vi "Basic.vi"() -> ()   [LabVIEW 2021, in "GettingStarted_5745_Host.lvlib"]
uses:
  GettingStarted_5745_Host.lvlib
  <vilib>/userdefined/High Color/nirio_resource_hc.ctl
  <instrlib>/FlexRIO/API/Host/v1/NI FlexRIO/API/Reference Clock Source.ctl
  <vilib>/rvi/interface/common/niFpgaWaitOnOcc.vi
  <vilib>/Utility/error.llb/Error Cluster From Error Code.vi
  <instrlib>/FlexRIO/API/Host/v1/NI FlexRIO/API/Configure Reference Clock.vi
  <instrlib>/FlexRIO/API/Host/v1/NI FlexRIO/API/Configure Digital Edge Start Trigger.vi
  <instrlib>/FlexRIO/API/Host/v1/NI FlexRIO/API/Configure Immediate Start Trigger.vi
  <instrlib>/_niInstr/Streaming/v1/Host/Public/Start Continuous Stream.vi
  <vilib>/FPGAPlugInAG/Dynamic/niLvFpga_Close_Dynamic.vi
  <vilib>/rvi/interface/nirviMethod/nirviMethod.xnode
  <vilib>/rvi/interface/nirviCloseFPGA/nirviCloseFPGA.xnode
  <instrlib>/FlexRIO/API/Host/v1/NI FlexRIO API v1.lvlib
  <instrlib>/_niInstr/Streaming/v1/Host/niInstr Streaming v1 Host.lvlib
  <vilib>/FPGAPlugInAG/Dynamic/niLvFpga_ConfigureFifo_Dynamic.vi
  <vilib>/rvi/errors/niLvFpgaMergeErrorWithErrorCode.vi
panel:
  in  "reference clock source":T1 items=["Default", "Onboard", "PXI_Clk10", "External", "None", "Baseboard Reference"]
  in  "Download AO Waveforms":bool
  out "AO Out":waveform(dbl)[](graph) caption="Waveform Graph"
  in  "Phase (Deg)":dbl format="%.2p"
  in  "Phase (Deg) 2":dbl=-90.0 format="%.2p"
  in  "Enable DAC Digital Upconverter":bool
  in  "DAC Digital Upconverter Channel":string="AO0"
  in  "Amplitude (V)":dbl=0.4 format="%0.2p"
  in  "Frequency (Hz)":dbl=5000000.0 format="%0.2p"
  in  "Amplitude (V) 2":dbl=0.4 format="%0.2p"
  in  "Frequency (Hz) 2":dbl=10000000.0 format="%0.2p"
  in  "Sampling Info":cluster{"Fs":dbl, "#s":dbl}={"Fs"=3200000000.0, "#s"=3200.0} {"#s" format="%_9g"; "Fs" format="%#_6p"}
  out "Device Power":dbl(slide)=17.86 scale=-1.0..38.0 scale format="%#_3p"
  out "FPGA Temperature":dbl(slide)=45.0 scale=0.0..100.0 scale format="%#_3p"
  in  "Trigger Type":enum32{"Immediate", "Digital"}(tab)
  in  "digital trigger source":string(combo)
  in  "stop":bool
  in  "Bitfile path":path=path "C:/Program Files (x86)/National Instruments/LabVIEW 2022/ProjectTemplates/Source/FlexRIO/NI5745/Getting Started/FPGA Bitfiles/PXIe_5745_KU040.lvbitx"
  out "error out":errorcluster
  out "Limit (W)":dbl=38.0
  out "Power (W)":dbl=17.86
  out "Limit (C)":dbl=96.0
  out "Temp (C)":dbl=45.0 format="%#_4p"
  in  "RIO Device":T2="5745_1"
  # "Overview: Configure an acquisition for a FlexRIO target and transfer the data to the host using the FlexRIO Host API.  Loop an output waveform\nRequirements: FlexRIO\nInstructions: \n 1. Select the RIO Device that corresponds to the FlexRIO target. \n 2. Select the bitfile path that corresponds to your device\n 3. Optionally configure the clocking, stream, and trigger. \n 4. Run the VI"
  # "Resource Configuration"
  # "Clocking configuration"
  # "25600.0000\n22400"
  # "Output Waveform Configuration"
  # "Device Monitoring"
  # "AO 0"
  # "AO 1"
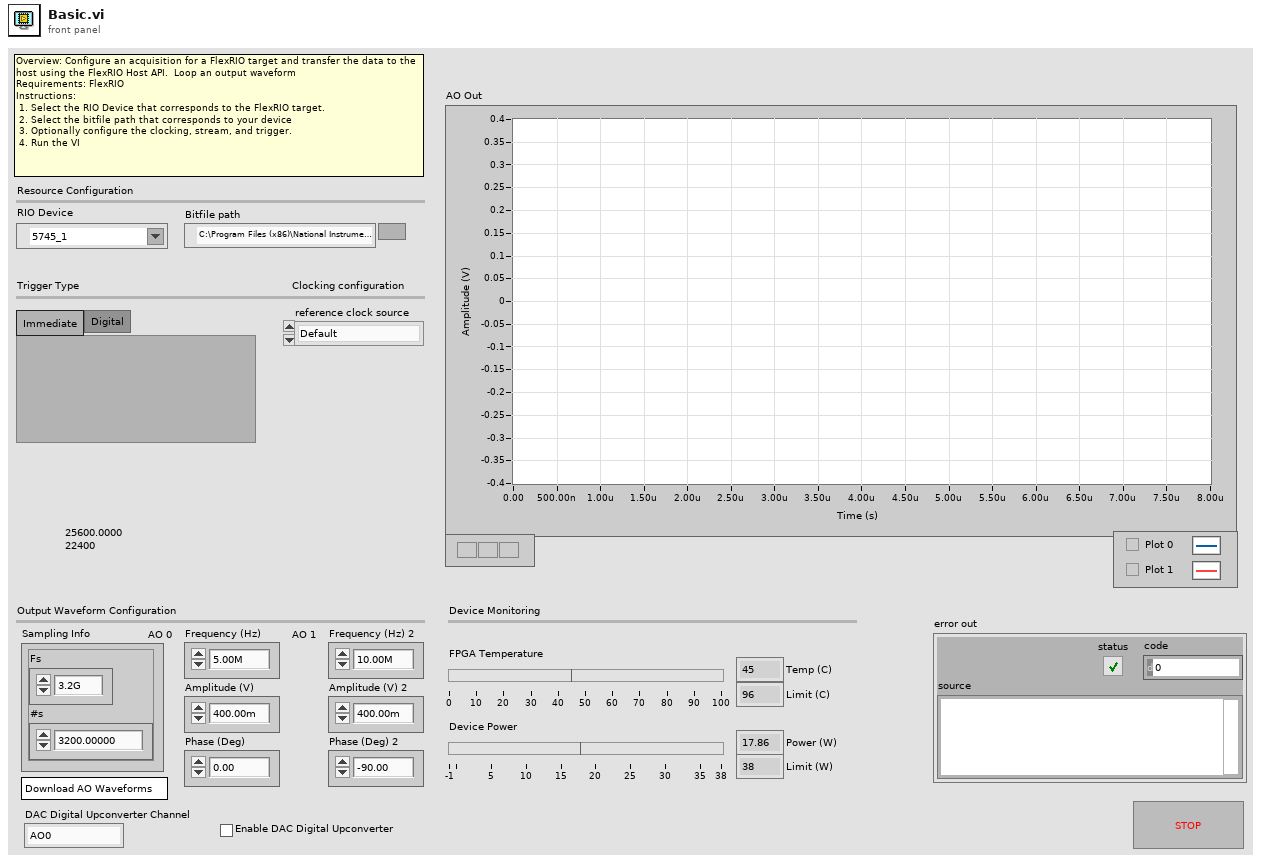
[diagram p1: front panel]
types:
  T1 = typedef "NI FlexRIO API v1.lvlib/Reference Clock Source.ctl" = i32
  T2 = typedef "nirio_resource_hc.ctl" = tag
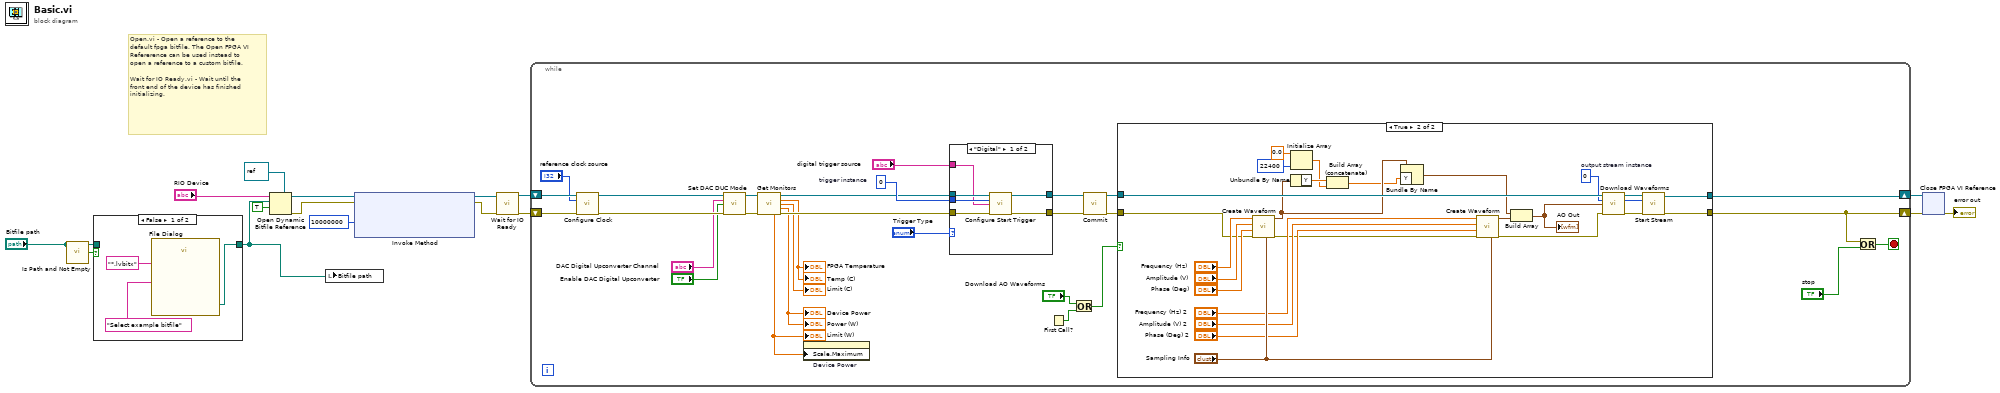
[diagram p0: block diagram]
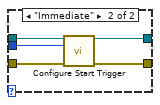
[diagram p3: hidden frame]
diagram:
  # "Open.vi - Open a reference to the default fpga bitfile. The Open FPGA VI Refererence can be used instead to open a reference to a custom bitfile.\n\nWait for IO Ready.vi - Wait until the front end of the device has finished initializing."
  n1 = call <vilib>:"Is Path and Not Empty.vi"("path"="Bitfile path") -> ("Is Path and Not Empty?"=w7:bool)  [unwired: 4 in]
  n2 = case shown="False" w7 {
    tunnel: "Bitfile path" -> [_ w20]
    tunnel: [w18 w20] -> w6
    frame False {
      n3 = call "File Dialog"("prompt"="Select example bitfile", "pattern (all files)"="*.lvbitx") -> ("selected path"=w18:path)  [unwired: 10 in, 3 out]
    }
    frame True {
    }
  }
  n4 = Open Dynamic Bitfile Reference(0:"RIO Device", 1:w6, 2:TRUE ("Run When Loaded"), 4:refnum<k20> refnum ("Type")) -> (5:w13:refnum<k20>, 8:w3:errorcluster)  [unwired: 1 in]
  n5 = local write "Bitfile path"(w6) -> ()
  n6 = xnode "Invoke Method"("FPGA VI Reference In"=w13, "error in"=w3, "Requested Depth"=u32 10000000) -> ("FPGA VI Reference Out"=w5:refnum<k20>, "error out"=w2:errorcluster)  [unwired: 1 out]
  n7 = call <instrlib>:"Wait for IO Ready.vi"("fpga interface in"=w5, "error in"=w2) -> ("fpga interface out"=w14:refnum<k20>, "error out"=w15:errorcluster)  [unwired: 10 in, 2 out]
  n8 = while {
    shift-right: [w38] -> w9
    shift-left: w15 -> [w45]
    shift-right: [w39] -> w10
    shift-left: w14 -> [w44]
    stop <- w35 stop-if-true
    w46 = u32 0  # trigger instance
    n9 = call-poly <instrlib>:"Configure Clock.vi"("fpga interface in"=w44, "reference clock source"="reference clock source", "error in"=w45) -> ("fpga interface out"=w49:refnum<k20>, "error out"=w48:errorcluster)  [unwired: 11 in]
    n10 = call "Set DAC DUC Mode.vi"("fpga interface in"=w49, "DAC Digital Upconverter Channel"="DAC Digital Upconverter Channel", "Enable DAC Digital Upconverter"="Enable DAC Digital Upconverter", "error in (no error)"=w48) -> ("fpga interface out"=w33:refnum<k20>, "error out"=w34:errorcluster)  [unwired: 10 in]
    n11 = call "Get Monitors.vi"("fpga interface in"=w33, "error in (no error)"=w34) -> ("fpga interface out"=w30:refnum<k20>, "FPGA Temperature (C)"=→"Temp (C)" →"FPGA Temperature":dbl, "Temperature Limit (C)"=→"Limit (C)":dbl, "Total Power (W)"=→"Power (W)" →"Device Power":dbl, "Power Limit (W)"=w26:dbl, "error out"=w31:errorcluster)  [unwired: 8 in]
    "Limit (W)" <- w26
    n12 = property on="Device Power" class="Slide (strict)"("Scale.Maximum"=w26) -> ()  [unwired: 2 in, 2 out]
    n13 = case shown="\"Digital\"" "Trigger Type" {
      tunnel: w30 -> [w83 w88]
      tunnel: w31 -> [w82 w87]
      tunnel: [w81 w86] -> w42
      tunnel: [w80 w85] -> w41
      tunnel: w46 -> [w79 w84]
      tunnel: "digital trigger source" -> [w78 _]
      frame "Digital" {
        n14 = call-poly <instrlib>:"Configure Start Trigger.vi"("fpga interface in"=w83, "trigger instance"=w79, "trigger source"=w78, "error in"=w82) -> ("fpga interface out"=w81:refnum<k20>, "error out"=w80:errorcluster)  [unwired: 9 in, 1 out]
      }
      frame "Immediate" {
        n15 = call-poly <instrlib>:"Configure Start Trigger.vi"("fpga interface in"=w88, "trigger instance"=w84, "error in"=w87) -> ("fpga interface out"=w86:refnum<k20>, "error out"=w85:errorcluster)  [unwired: 10 in, 1 out]
      }
    }
    n16 = First Call?() -> (First Call?: T/F=w23:bool)
    n17 = Or(x="Download AO Waveforms", y=w23) -> (x .or. y?=w22:bool)
    n18 = call <instrlib>:"Commit.vi"("fpga interface in"=w42, "error in"=w41) -> ("fpga interface out"=w43:refnum<k20>, "error out"=w37:errorcluster)  [unwired: 12 in]
    n19 = case shown="True" w22 {
      tunnel: w43 -> [w51 w70]
      tunnel: [w51 w64] -> w39
      tunnel: [w50 w63] -> w38
      tunnel: w37 -> [w50 w61]
      frame False {
      }
      frame True {
        w67 = 0  # output stream instance
        n20 = call "Create Waveform.vi"("sampling info"="Sampling Info", "error in (no error)"=w61, "phase"="Phase (Deg)", "amplitude"="Amplitude (V)", "frequency"="Frequency (Hz)") -> ("error out"=w59:errorcluster, "Output Waveform (V)"=w54:waveform(dbl))  [unwired: 4 in, 1 out]
        n21 = Initialize Array(0.0 ("element"), 22400 ("dimension size")) -> (w55:dbl[])
        n22 = Unbundle By Name(w54) -> ("Y"=w56:dbl[])
        n23 = Build Array (concatenate)(w56, w55) -> (w53:dbl[])
        n24 = Bundle By Name(cluster=w54, "Y"=w53) -> (w52:waveform(dbl))
        n25 = call "Create Waveform.vi"("sampling info"="Sampling Info", "error in (no error)"=w59, "phase"="Phase (Deg) 2", "amplitude"="Amplitude (V) 2", "frequency"="Frequency (Hz) 2") -> ("error out"=w60:errorcluster, "Output Waveform (V)"=w62:waveform(dbl))  [unwired: 4 in, 1 out]
        n26 = Build Array(w52, w62) -> (w65:waveform(dbl)[])
        "AO Out" <- w65
        n27 = call "Download Waveforms.vi"("fpga interface in"=w70, "stream instance"=w67, "waveforms"=w65, "error in"=w60) -> ("fpga interface out"=w76:refnum<k20>, "stream instance out"=w66:i32, "error out"=w75:errorcluster)  [unwired: 9 in]
        n28 = call-poly <instrlib>:"Start Stream.vi"("error in (no error)"=w75, "stream index"=w66, "refnum in"=w76) -> ("error out"=w63:errorcluster, "refnum out"=w64:refnum<k20>)  [unwired: 7 in]
      }
    }
    n29 = Or(x=w38, y="stop") -> (x .or. y?=w35:bool)
  }
  n30 = xnode "Close FPGA VI Reference"("FPGA VI Reference In"=w10, "error in"=w9) -> ("error out"=→"error out":errorcluster)
